vi "Destroy.vi"(0 "reference in":refnum<class "OffensivePlay.lvclass">, 5 "error in (no error)":errorcluster) -> (14 "reference out":refnum<class "OffensivePlay.lvclass">, 19 "error out":errorcluster)   [LabVIEW 2018, in "OffensivePlay.lvclass"]
uses:
  OffensivePlay.lvclass
  Play_class/Play.lvclass
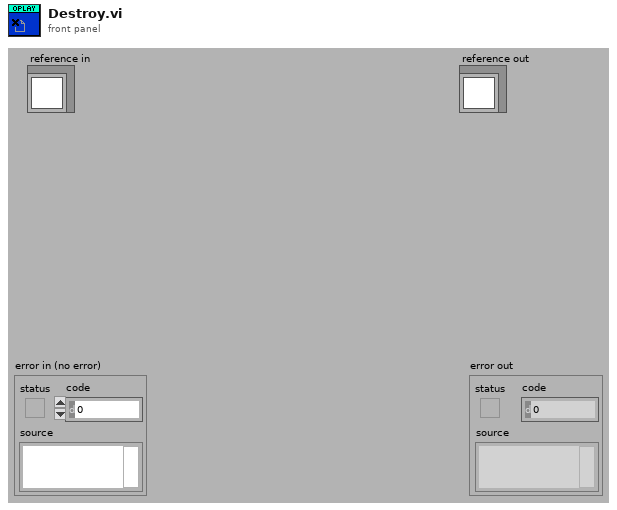
[diagram p1: front panel]
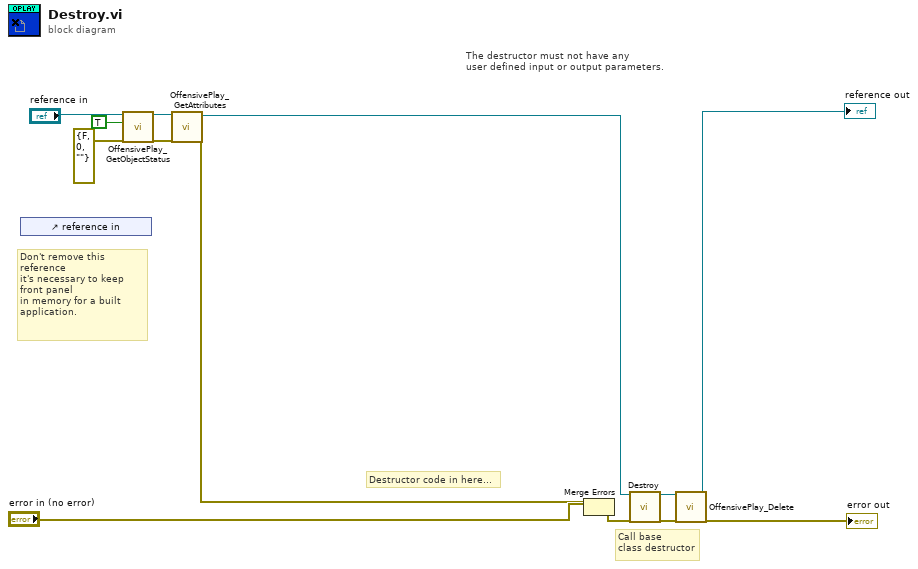
[diagram p0: block diagram]
diagram:
  # "Don't remove this reference\nit's necessary to keep front panel\nin memory for a built application."
  # "Destructor code in here..."
  # "The destructor must not have any\nuser defined input or output parameters."
  # "Call base\nclass destructor"
  n1 = control-ref of="reference in"() -> ()  [unwired: 1 out]
  n2 = call "OffensivePlay_GetObjectStatus.vi"("reference in"="reference in", "Simple Info"=TRUE, "error in (no error)"=errorcluster {"status"=FALSE, "code"=0, "source"=""}) -> ("reference out"=w5:refnum<class "OffensivePlay.lvclass">, "error out"=w3:errorcluster)  [unwired: 6 in, 9 out]
  n3 = call "OffensivePlay_GetAttributes.vi"("reference in"=w5, "error in (no error)"=w3) -> ("reference out"=w9:refnum<class "OffensivePlay.lvclass">, "error out"=w6:errorcluster)  [unwired: 14 in, 2 out]
  n4 = Merge Errors("error in (no error)", w6) -> (w12:errorcluster)
  n5 = call-parent "Destroy.vi"("reference in"=w9, "error in (no error)"=w12) -> ("reference out"=w8:refnum<class "OffensivePlay.lvclass">, "error out"=w11:errorcluster)  [unwired: 16 in]
  n6 = call "OffensivePlay_Delete.vi"("reference in"=w8, "error in (no error)"=w11) -> ("reference out"=→"reference out":refnum<class "OffensivePlay.lvclass">, "error out"=→"error out":errorcluster)  [unwired: 15 in, 1 out]
